vi "Clear GUI Errors.vi"(8 "error in (no error)":errorcluster, 11 "Alarm Handler Actor in":refnum<class "Alarm Handler Actor.lvclass">) -> (0 "error out":errorcluster, 3 "Alarm Handler Actor out":refnum<class "Alarm Handler Actor.lvclass">)   [LabVIEW 2015, in "Alarm Handler Actor.lvclass"]
uses:
  Alarm Handler Actor.lvclass
  Alarm Handler Actor.lvclass/Alarm Handler Actor.ctl
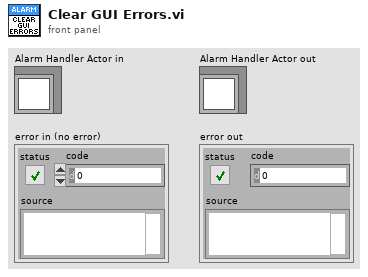
[diagram p1: front panel]
types:
  T1 = typedef "Alarm Handler Actor.lvclass/Active Alarm.ctl" = cluster{"Alarm Detail":T2, "Count":i32, "First Error":timestamp, "Last Error":timestamp, "LabVIEW Error":bool}
  T2 = typedef "Alarm Handler Actor.lvclass/Alarm Details.ctl" = cluster{"Code":i32, "Loop":i32, "Description":string, "Severity":i32, "Clear on Ack?":bool, "Log All Events?":bool}
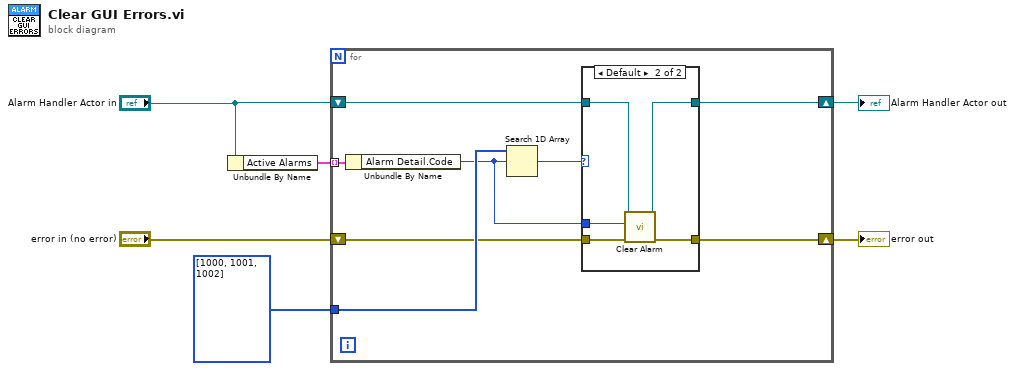
[diagram p0: block diagram]
diagram:
  n1 = Unbundle By Name("Alarm Handler Actor in") -> ("Active Alarms"=w6:T1[])
  n2 = for {
    shift-right: [w11] -> w2
    shift-left: "Alarm Handler Actor in" -> [w12]
    shift-right: [w9] -> w3
    shift-left: "error in (no error)" -> [w8]
    tunnel: i32[] [1000, 1001, 1002] -> [w13]
    tunnel: w6 -> [w14] mode=indexing
    n3 = Unbundle By Name(w14) -> ("Alarm Detail.Code"=w7:i32)
    n4 = Search 1D Array(1D array=w13, element=w7) -> (index of element=w10:i32)  [unwired: 1 in]
    n5 = case shown="Default" w10 {
      tunnel: w12 -> [w16 w21]
      tunnel: [w16 w20] -> w11
      tunnel: [w15 w18] -> w9
      tunnel: w8 -> [w15 w19]
      tunnel: w7 -> [_ w17]
      frame -1 {
      }
      frame Default {
        n6 = call "Clear Alarm.vi"("error in (no error)"=w19, "Alarm Code"=w17, "Alarm Handler Actor in"=w21) -> ("error out"=w18:errorcluster, "Alarm Handler Actor out"=w20:refnum<class "Alarm Handler Actor.lvclass">)  [unwired: 7 in]
      }
    }
  }
  "Alarm Handler Actor out" <- w2
  "error out" <- w3
